vi "Replace date by add 1 in date from time stamp.vi"(7 "Current Date":timestamp, 11 "Time Stamp in":timestamp=timestamp(3597613200 s since 1904-01-01)) -> (3 "Time Stamp Out":timestamp=timestamp(3597613200 s since 1904-01-01))   [LabVIEW 2017]
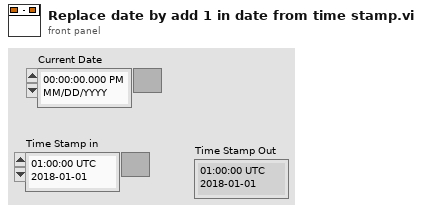
[diagram p1: front panel]
types:
  T1 = typedef "LVDateTimeRec.ctl" = cluster{"fractional second":dbl, "second":i32, "minute":i32, "hour":i32, "day of month":i32, "month":i32, "year":i32, "day of week":i32, "day of year":i32, "DST":i32}
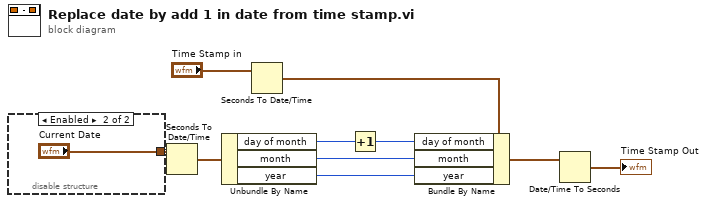
[diagram p0: block diagram]
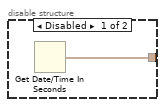
[diagram p2: hidden frame]
diagram:
  n1 = disable-structure shown="Enabled" {
    disable-tunnel: [w11 "Current Date"] -> w9
    frame Disabled {
      n2 = Get Date/Time In Seconds() -> (seconds since 1Jan1904=w11:timestamp)
    }
    frame Enabled {
    }
  }
  n3 = Seconds To Date/Time(time stamp (now)=w9) -> (date time rec=w8:T1)  [unwired: 1 in]
  n4 = Unbundle By Name(w8) -> ("day of month"=w6:i32, "month"=w5:i32, "year"=w4:i32)
  n5 = Seconds To Date/Time(time stamp (now)="Time Stamp in") -> (date time rec=w7:T1)  [unwired: 1 in]
  n6 = Increment(x=w6) -> (x+1=w1:i32)
  n7 = Bundle By Name(cluster=w7, "day of month"=w1, "month"=w5, "year"=w4) -> (w3:T1)
  n8 = Date/Time To Seconds(2:w3) -> (0:→"Time Stamp Out":timestamp)  [unwired: 1 in]
